vi "Test DIO.vi"() -> ()   [LabVIEW 2015]
uses:
  <vilib>/DAQmx/create/channels.llb/DAQmx Create Channel (DO-Digital Output).vi
  <vilib>/DAQmx/write.llb/DAQmx Write (Digital 2D Bool NChan 1Samp NLine).vi
  <vilib>/DAQmx/read.llb/DAQmx Read (Digital 2D Bool NChan 1Samp NLine).vi
panel:
  out "DO":string
  out "data read":bool[][](array[boolean])
  in  "data":bool[][](array[boolean])
  out "number of samples written per channel":u32
  in  "stop":bool
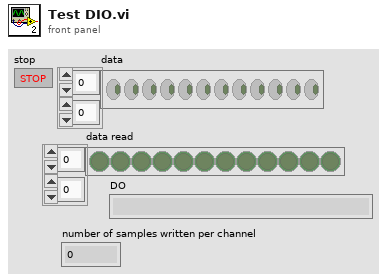
[diagram p1: front panel]
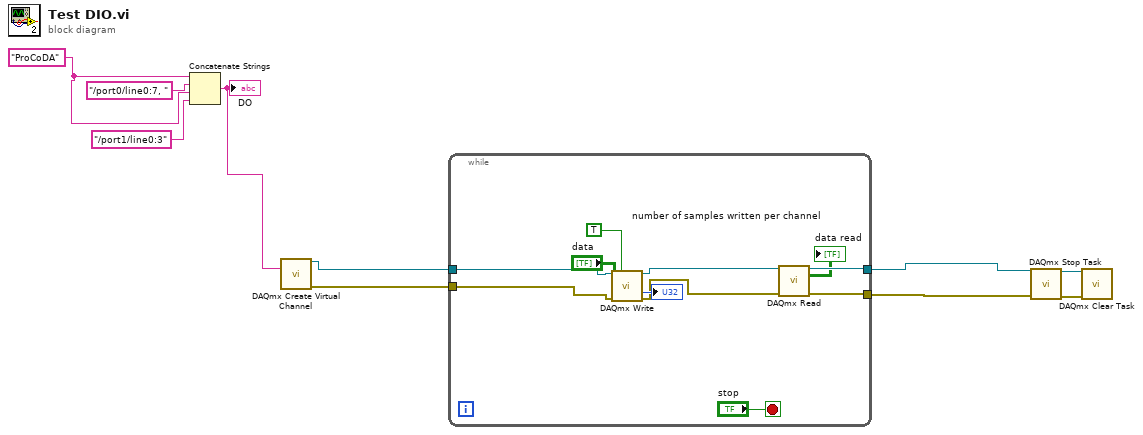
[diagram p0: block diagram]
diagram:
  w2 = "ProCoDA" ("string")
  n1 = Concatenate Strings(w2, "/port0/line0:7, ", w2, "/port1/line0:3") -> (w1:string)
  "DO" <- w1
  n2 = call-poly <vilib>:"DAQmx Create Virtual Channel.vi"("lines"=w1) -> ("task out"=w10:refnum<k21>, "error out"=w9:errorcluster)  [unwired: 13 in]
  n3 = while {
    tunnel: w10 -> [w19]
    tunnel: w9 -> [w20]
    tunnel: [w14] -> w5
    tunnel: [w12] -> w6
    stop <- "stop" stop-if-true
    n4 = call-poly <vilib>:"DAQmx Write.vi"("task/channels in"=w19, "auto start"=TRUE, "data"="data", "error in"=w20) -> ("task out"=w15:refnum<k21>, "number of samples written per channel"=→"number of samples written per channel":u32, "error out"=w13:errorcluster)  [unwired: 9 in]
    n5 = call-poly <vilib>:"DAQmx Read.vi"("task/channels in"=w15, "error in"=w13) -> ("task out"=w14:refnum<k21>, "data"=→"data read":bool[][], "error out"=w12:errorcluster)  [unwired: 11 in]
  }
  n6 = call <vilib>:"DAQmx Stop Task.vi"("task/channels in"=w5, "error in"=w6) -> ("task out"=w8:refnum<k21>, "error out"=w7:errorcluster)  [unwired: 12 in]
  n7 = call <vilib>:"DAQmx Clear Task.vi"("task in"=w8, "error in"=w7) -> ()  [unwired: 13 in, 1 out]
